vi "Initialize.vi"(7 "TimingEngine":T1, 8 "error in (no error)":errorcluster, 10 "Chassis Cfg":refnum<class "ChassisCfg.lvclass">, 11 "Chassis Name":string) -> (0 "error out":errorcluster, 2 "Num of Chans":i32, 3 "DAQ Task out":refnum<class "DAQ Task.lvclass">)   [LabVIEW 2018, in "Data Acquisition.lvlib" / "DAQ Task.lvclass"]
uses:
  DAQ Task.lvclass
  Common/Controls/TE_Designator.ctl
  Cfg Grandmaster/Class Chassis Cfg/ChassisCfg.lvclass
  Cfg Grandmaster/Class Chassis Cfg/ChassisCfg.lvclass/ChassisCfg.ctl
  DAQ Task.lvclass/DAQ Task.ctl
  Cfg Grandmaster/Class Chassis Cfg/Read Timing Grps.vi
  Cfg Grandmaster/Class Timing Group/TimingGrp.lvclass
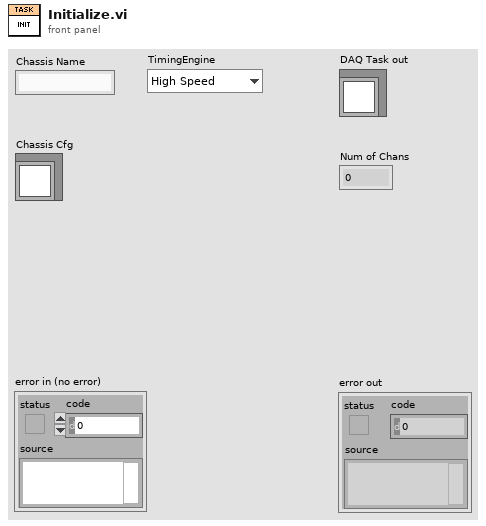
[diagram p1: front panel]
types:
  T1 = typedef "TE_Designator.ctl" = enum16{"High Speed", "Low Speed"}
  T2 = typedef "Group Timing Info.ctl" = cluster{"Rate":dbl, "ReadBlk":i32}
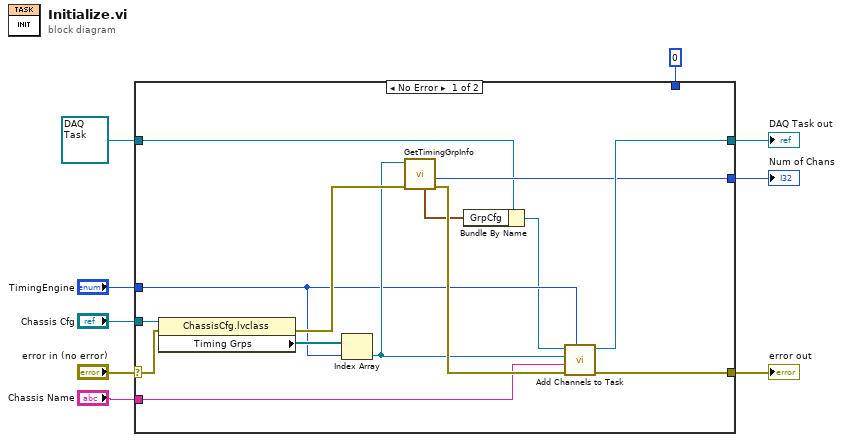
[diagram p0: block diagram]
diagram:
  n1 = case shown="No Error" "error in (no error)" {
    selector: "error in (no error)" -> [w18 w26]
    tunnel: [w23 w26] -> w8
    tunnel: [w22 w25] -> w6
    tunnel: refnum<class "DAQ Task.lvclass"> refnum ("DAQ Task in") -> [w12 w25]
    tunnel: "TimingEngine" -> [w13 _]
    tunnel: "Chassis Name" -> [w14 _]
    tunnel: "Chassis Cfg" -> [w19 _]
    tunnel: [w20 w24] -> w2
    tunnel: 0 ("Num of Chans") -> [_ w24]
    frame No Error {
      n2 = property class="ChassisCfg.lvclass"(reference=w19, error in=w18) -> (error out=w17:errorcluster, "Timing Grps"=w16:refnum<class "TimingGrp.lvclass">[])  [unwired: 1 out]
      n3 = Index Array(array=w16, index=w13) -> (element=w15:refnum<class "TimingGrp.lvclass">)
      n4 = call "GetTimingGrpInfo.vi"("error in"=w17, "TimingGrp in"=w15) -> ("error out"=w21:errorcluster, "Num of Chans"=w20:i32, "Timing Cfg"=w10:T2)  [unwired: 4 in, 3 out]
      n5 = Bundle By Name(cluster=w12, "GrpCfg"=w10) -> (w11:refnum<class "DAQ Task.lvclass">)
      n6 = call "Add Channels to Task.vi"("TimingEngine"=w13, "error in"=w21, "Chassis Name"=w14, "Timing Grp"=w15, "DAQ Task"=w11) -> ("error out"=w23:errorcluster, "DAQ Task"=w22:refnum<class "DAQ Task.lvclass">)  [unwired: 5 in]
    }
    frame Error {
    }
  }
  "error out" <- w8
  "DAQ Task out" <- w6
  "Num of Chans" <- w2
